vi "Dashboard Main.vi"() -> ()   [LabVIEW 2013]
uses:
  <vilib>/event_ctls.llb/eventvkey.ctl
  <vilib>/Rock Robotics/WPI/Dashboard/WPI_DashboardLogging Global.vi
  <vilib>/Utility/config.llb/Write Key (String).vi
  <vilib>/Utility/config.llb/Write Key (I32).vi
  <vilib>/Utility/config.llb/NI_LVConfig.lvlib
panel:
  out "LED 1":bool
  out "Image Message":string="Timeout in Camera Communications"
  in  "Rec Mode":enum32{"Stop", "Record", "Playback"}(radio)
  in  "Dashboard Tab":T1(tab)
  out "Re-Capture":bool
  out "Ping":dbl
  out "Gauge":dbl(knob) scale=0.0..180.0
  in  "1":dbl=1.0 min=1.0 max=3.0 step=1.0
  in  "Camera Settings":T2={"Frame Rate"=30, "Compression"=30, "Size"=1} {"Frame Rate" scale=1.0..30.0; "Size" items=["640x480", "320x240", "160x120"]}
  out "MotorSliders R":cluster{"MotorSlide1":dbl, "MotorSlide2":dbl} {"MotorSlide2" scale=-1.0..1.0 scale format="%#_2e"; "MotorSlide1" scale=-1.0..1.0 scale format="%#_2e"}
  out "MotorChart R":cluster{"Numeric":dbl, "Numeric":dbl}(graph)
  out "MotorSliders L":T3 {"MotorSlide4 2" scale=0.0..14.0 scale format="%#_2e"; "MotorSlide2" scale=-1.0..1.0 scale format="%#_2e"; "MotorSlide1" scale=-1.0..1.0 scale format="%#_2e"}
  out "MotorChart L":T4(graph)
  out "JS1 Z":dbl(slide) scale=-1.0..1.0 scale format="%#_2e"
  out "Joystick 1":cluster{"X":dbl, "Y":dbl}[](graph)
  out "JS Buttons 1":T5
  out "JS2 Z":dbl(slide) scale=-1.0..1.0 scale format="%#_2e"
  out "Joystick 2":cluster{"X":dbl, "Y":dbl}[](graph)
  out "JS Buttons 2":T5
  out "Mode":T6(ring)=enum."Auto Disabled"
  out "Camera IP":string
  in  "DB Camera Config":bool
  out "fps":dbl format="%#.1g"
  out "Mbps":dbl format="%#.1g"
  out "Mbps 2":bool
  out "Ready to Fire":bool
  out "Vacuum State":bool
  out "Manual":bool
  out "1":bool
  out "2":bool
  out "3":bool
  out "4":bool
  out "Blink":dbl
  out "Ticks":dbl
  out "State Machine State":dbl
  out "State Machine State Name":string
  in  "Slider 1":dbl(slide) scale=0.0..100.0
  in  "Checkbox 2":bool
  in  "Checkbox 1":bool
  in  "Test Slider":dbl(slide) scale=0.0..100.0 scale format="%#_3g"
  in  "On/Off":bool caption="Solenoid"
  in  "Test Name":u16(ring) items=["Select the test to run...", "Example Test", "-------------------------------", "List of tests is built in robot code.", "Replace with your own automated tests."]
  in  "Test Tree":string(tree)
  in  "Motor":cluster{"Value":dbl, "Enable":bool} {"Value" scale=-1.0..1.0 scale format="%#_3g"}
  out "Progress":T7 {"Test Progress" scale=0.0..100.0}
  in  "Rev/Fwd":cluster{"Forward":bool, "Reverse":bool}
  in  "Test Ring":u16(ring) items=["Auto", "Fixed indoor", "Fixed outdoor 1", "Fixed outdoor 2", "Fixed fluorescent 1", "Fixed fluorescent 2", "Hold current"]
  in  "Listbox":i32(listbox)
  out "Tree":string(tree)
  out "Camera Image":T8(plugin-control)
  in  "Enable":bool
  # "Autonomous Presets"
  # "Left"
  # "Front"
  # "Right"
  # "Battery"
  # "Customize by placing controls and indicators here and name to\nmatch Dashboard Variables on robot."
  # "This tab is a great place for autonomous settings and validation.\nCustomize by placing controls and indicators here and name to\nmatch Dashboard Variables on robot."
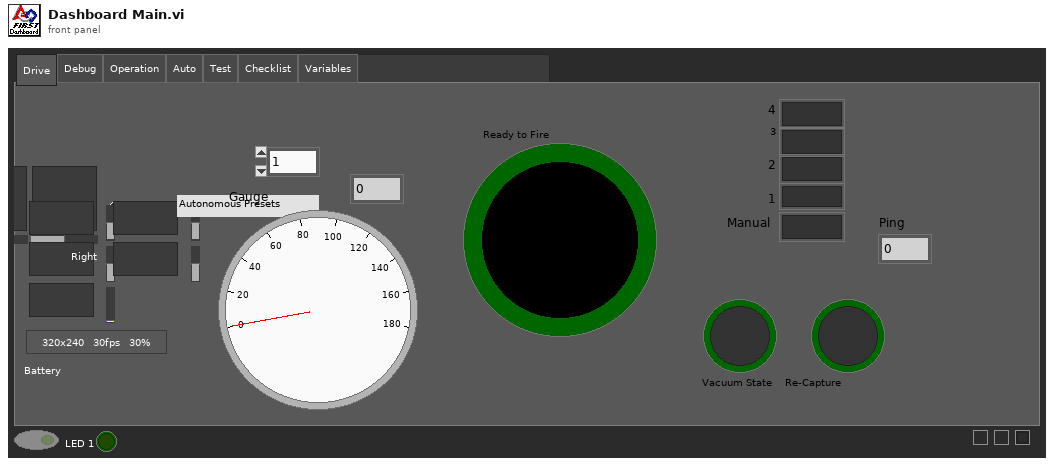
[diagram p1: front panel]
types:
  T1 = enum32{"Drive", "Debug", "Operation", "Auto", "Test", "Checklist", "Variables"}
  T2 = cluster{"Frame Rate":i32, "Compression":i32, "Size":u16}
  T3 = cluster{"MotorSlide1":dbl, "MotorSlide2":dbl, "MotorSlide4 2":dbl}
  T4 = cluster{"Numeric":dbl, "Numeric":dbl, "Battery":sgl}
  T5 = cluster{bool, bool, bool, bool, bool, bool, bool, bool, bool, bool, bool, bool}
  T6 = enum8{"Tele-Op Disabled", "Tele-Op Enabled", "Auto Disabled", "Auto Enabled", "Test Disabled", "Test Enabled", ""}
  T7 = cluster{"Test Progress":u8, "Test Progress Text":string}
  T8 = typedef "IMAQ Image.ctl" = refnum<image>
  T9 = enum32{"Drive", "Operation", "Auto", "Test", "Checklist", "Variables"}
  T10 = typedef "Image Type" = u32
  T11 = cluster{"Digital Inputs":bool[], "Digital Outputs":bool[]}
  T12 = cluster{"Competition mode":bool, "Robot Link":bool, "Autonomous":bool, "Enabled":bool, "E-Stop":bool, "Simulated":bool, "TestMode":bool, "Docked Window":bool}
  T13 = cluster{"Boolean Array[0]":bool, "Boolean Array[1]":bool, "Boolean Array[2]":bool, "Boolean Array[3]":bool, "Boolean Array[4]":bool, "Boolean Array[5]":bool, "Boolean Array[6]":bool, "Boolean Array[7]":bool, "Boolean Array[8]":bool, "Boolean Array[9]":bool, "Boolean Array[10]":bool, "Boolean Array[11]":bool}
  T14 = typedef "NI_LVConfig.lvlib/Config Data RefNum.ctl" = refnum<k1>
  T15 = typedef "eventvkey.ctl" = enum16{"ASCII", "Enter", "Return", "Shift", "Ctrl", "Alt", "Cmd", "Opt", "Caps", "NumLock", "Clear", "Break", "Up", "Down", "Left", "Right", "Insert", "Delete", "Home", "End", "PageUp", "PageDown", "Escape", "Help", "Pause", "ScrollLock", "F1", "F2", "F3", "F4", "F5", "F6", "F7", "F8", "F9", "F10", "F11", "F12", "F13", "F14", "F15", "F16", "F17", "F18", "F19", "F20", "F21", "F22", "F23", "F24", "Play", "VolumeUp", "VolumeDown", "Mute", "Two Byte Char"}
  T16 = cluster{"Image Size":bool, "Image Type":bool, "Pixel Value":bool, "ROI Information":bool, "Zoom Factor":bool}
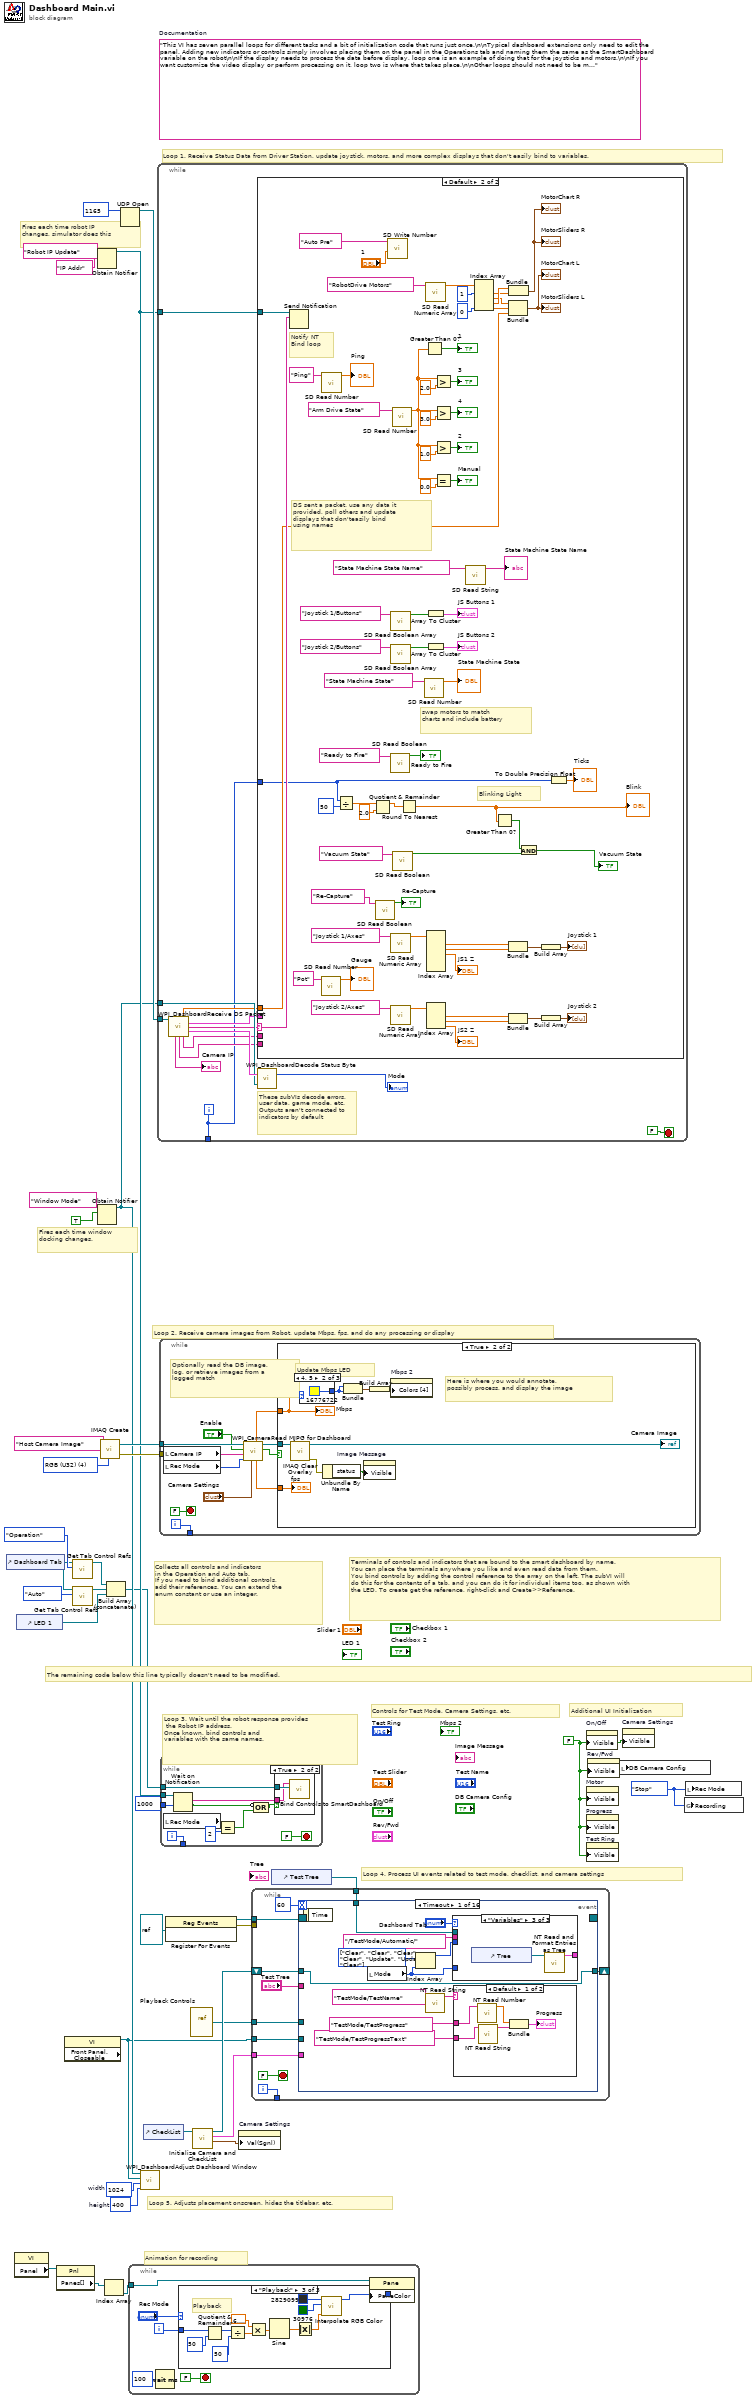
[diagram p0: block diagram]
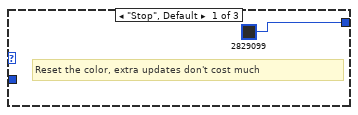
[diagram p2: hidden frame]
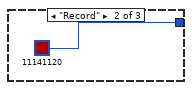
[diagram p3: hidden frame]
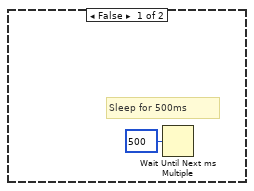
[diagram p5: hidden frame]
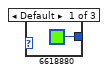
[diagram p6: hidden frame]
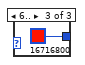
[diagram p7: hidden frame]
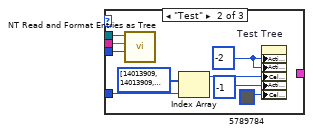
[diagram p9: hidden frame]
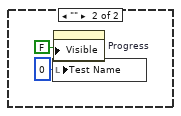
[diagram p10: hidden frame]
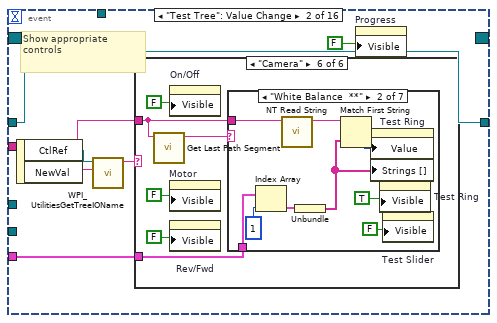
[diagram p11: hidden frame]
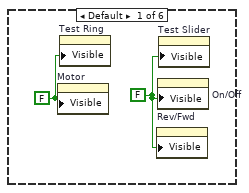
[diagram p12: hidden frame]
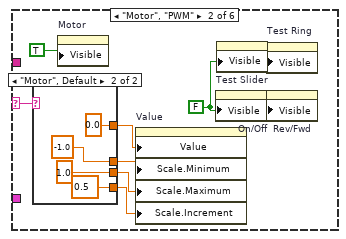
[diagram p13: hidden frame]
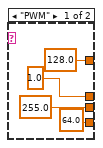
[diagram p14: hidden frame]
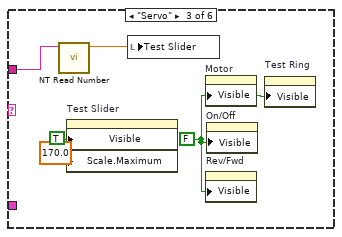
[diagram p15: hidden frame]
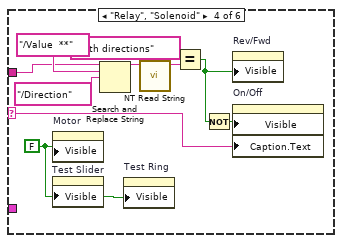
[diagram p16: hidden frame]
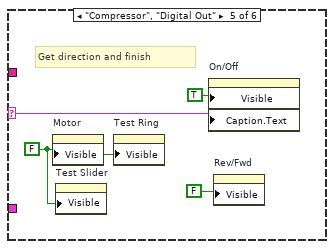
[diagram p17: hidden frame]
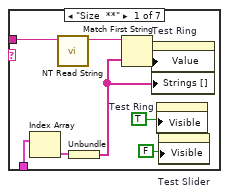
[diagram p18: hidden frame]
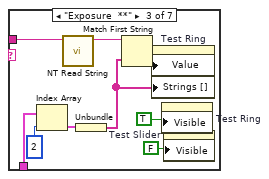
[diagram p19: hidden frame]
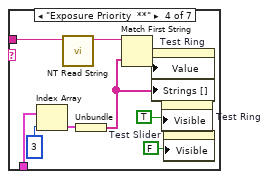
[diagram p20: hidden frame]
diagram:
  w8 = enum32{"Stop", "Record", "Playback"}."Stop" ("Rec Mode")
  w11 = 400  # height
  w12 = 1024  # width
  w25 = FALSE ("Visible")
  (unwired) "This VI has seven parallel loops for different tasks and a bit of initialization code that runs just once.\n\nTypical dashboard extensions only need to edit the panel. Adding new indicators or controls simply involves placing them on the panel in the Operations tab and naming them the same as the SmartDashboard variable on the robot\n\nIf the display needs to process the data before display, loop one is an example of doing that for the joysticks and motors.\n\nIf you want customize the video display or perform processing on it, loop two is where that takes place.\n\nOther loops should not need to be modified. They are pretty standard, and document the task they perform."  # Documentation
  w35 = T10 4 items=["Grayscale (U8)", "Grayscale (I16)", "Grayscale (SGL)", "Complex (CSG)", "RGB (U32)", "HSL (U32)", "RGB (U64)"] ("Image Type")
  # "Controls for Test Mode, Camera Settings, etc."
  # "Additional UI Initialization"
  # "Animation for recording"
  # "Fires each time robot IP\nchanges, simulator does this"
  # "Fires each time window\ndocking changes."
  # "Collects all controls and indicators\nin the Operation and Auto tab.\nIf you need to bind additional controls,\nadd their references. You can extend the\nenum constant or use an integer."
  # "The remaining code below this line typically doesn't need to be modified."
  # "Loop 4. Process UI events related to test mode, checklist, and camera settings"
  # "Terminals of controls and indicators that are bound to the smart dashboard by name.\nYou can place the terminals anywhere you like and even read data from them.\nYou bind controls by adding the control reference to the array on the left. The subVI will\ndo this for the contents of a tab, and you can do it for individual items too, as shown with\nthe LED. To create get the reference, right-click and Create>>Reference."
  # "Loop 3. Wait until the robot response provides\n the Robot IP address.\nOnce known, bind controls and\nvariables with the same names."
  # "Loop 5. Adjusts placement onscreen, hides the titlebar, etc."
  # "Loop 1. Receive Status Data from Driver Station, update joystick, motors, and more complex displays that don't easily bind to variables."
  # "Loop 2. Receive camera images from Robot, update Mbps, fps, and do any processing or display"
  n1 = control-ref of="Dashboard Tab"() -> (w6:refnum<vi>)
  n2 = property class="VI"() -> ("Panel"=w19:refnum<vi>)  [unwired: 2 in, 2 out]
  n3 = control-ref of="LED 1"() -> (w1:refnum<vi>)
  n4 = property class="Pnl"(reference=w19) -> ("Panes[]"=w20:refnum<vi>[])  [unwired: 1 in, 2 out]
  n5 = property class="VI" props=["Front Panel.Closeable"]() -> (reference out=w7:refnum<vi>)  [unwired: 2 in, 2 out]
  n6 = call <vilib>:"Get Tab Control Refs.vi"("Page Index"=T9."Operation" ("Dashboard Tab"), "TabControl in"=w6) -> ("ControlsOnPage"=w4:refnum<vi>[])  [unwired: 9 in]
  n7 = call <vilib>:"Get Tab Control Refs.vi"("Page Index"=T9."Auto" ("Dashboard Tab"), "TabControl in"=w6) -> ("ControlsOnPage"=w5:refnum<vi>[])  [unwired: 9 in]
  n8 = Obtain Notifier(name (unnamed)="Robot IP Update", notification data type="IP Addr" ("name (unnamed)")) -> (notifier out=w29:refnum<notifier>)  [unwired: 2 in, 2 out]
  n9 = Obtain Notifier(name (unnamed)="Window Mode", notification data type=TRUE) -> (notifier out=w10:refnum<notifier>)  [unwired: 2 in, 2 out]
  n10 = call "IMAQ Create"("Image Name"="Host Camera Image", "Image Type"=w35) -> ("New Image"=w33:T8, "error out"=w32:errorcluster)  [unwired: 2 in, 1 out]
  n11 = Index Array(array=w20) -> (element=w18:refnum<vi>)  [unwired: 1 in]
  n12 = Build Array (concatenate)(w4, w5, w1) -> (w3:refnum<vi>[])
  n13 = UDP Open(11:u16 1165 ("port")) -> (port=w36:refnum<k16>)  [unwired: 2 in, 4 out]
  n14 = while {
    tunnel: w18 -> [w39]
    i -> [w42]
    stop <- FALSE stop-if-true
    n15 = Wait (ms)(milliseconds to wait=u32 100) -> ()  [unwired: 1 out]
    n16 = case shown="\"Playback\"" "Rec Mode" {
      tunnel: w42 -> [_ _ w57]
      tunnel: [u32 2829099 ("Base Color") u32 11141120 ("Target Color") w46] -> w38
      frame "Stop", Default {
        # "Reset the color, extra updates don't cost much"
      }
      frame "Record" {
      }
      frame "Playback" {
        # "Playback"
        n17 = Quotient & Remainder(x=w57, y=u32 50 ("milliseconds to wait")) -> (x-y*floor(x/y)=w53:u32)  [unwired: 1 out]
        n18 = Divide(x=w53, y=u32 50 ("milliseconds to wait")) -> (x/y=w50:dbl)
        n19 = Multiply(x=6.283185307179586, y=w50) -> (x*y=w55:dbl)
        n20 = Sine(x=w55) -> (sin(x)=w54:dbl)
        n21 = Absolute Value(x=w54) -> (abs(x)=w47:dbl)
        n22 = call "Interpolate RGB Color.vi"("Proportion"=w47, "Target Color"=u32 30976, "Base Color"=u32 2829099) -> ("Result Color"=w46:u32)  [unwired: 8 in]
      }
    }
    n23 = property class="Pane"(reference=w39, "PaneColor"=w38) -> ()  [unwired: 1 in, 2 out]
  }
  n24 = call <vilib>:"WPI_DashboardAdjust Dashboard Window.vi"("height"=w11, "width"=w12, "reference in"=w7, "Notifier in"=w10) -> ()  [unwired: 8 in]
  n25 = control-ref of="CheckList"() -> (w9:refnum<vi>)
  n26 = while {
    tunnel: w36 -> [w68]
    tunnel: w29 -> [w64]
    tunnel: w10 -> [w67]
    tunnel: [w58] -> _
    i -> [w58]
    stop <- FALSE stop-if-true
    # "These subVIs decode errors, user data, game mode, etc.\nOutputs aren't connected to indicators by default"
    n27 = call <vilib>:"WPI_DashboardReceive DS Packet.vi"("Recv Socket"=w68) -> ("Battery"=w59:sgl, "Driver Station"=w60:T11, "Robot IP Address"=w63:string, "Status"=w69:T12, "Camera IP Address"=→"Camera IP":string, "Low Priority User Data"=w62:string, "High Priority User Data"=w61:string)  [unwired: 1 in, 7 out]
    n28 = case shown="Default" w63 {
      selector: w63 -> [_ w117]
      tunnel: w64 -> [_ w118]
      tunnel: w62 -> [_ _]
      tunnel: w61 -> [_ _]
      tunnel: w60 -> [_ _]
      tunnel: w59 -> [_ w116]
      tunnel: w58 -> [_ w77]
      frame "0.0.0.0" {
        # "DS not sending packets, or no robot exists yet.\nDon't poll the variables"
      }
      frame Default {
        # "Blinking Light"
        # "Notify NT\nBind loop"
        # "DS sent a packet. use any data it\nprovided, poll others and update\ndisplays that don'teasily bind\nusing names"
        # "swap motors to match\ncharts and include battery"
        n29 = Send Notification(notification=w117, notifier=w118) -> ()  [unwired: 1 in, 2 out]
        n30 = call <vilib>:"SD Read Number.vi"("Name"="Pot") -> ("Numeric"=→"Gauge":dbl)  [unwired: 8 in, 2 out]
        n31 = call <vilib>:"SD Read Number.vi"("Name"="Ping") -> ("Numeric"=→"Ping":dbl)  [unwired: 8 in, 2 out]
        n32 = Divide(x=w77, y=50) -> (x/y=w79:dbl)
        n33 = Quotient & Remainder(x=w79, y=2.0) -> (x-y*floor(x/y)=w75:dbl)  [unwired: 1 out]
        n34 = call <vilib>:"SD Read Boolean.vi"("Name"="Re-Capture") -> ("Boolean"=→"Re-Capture":bool)  [unwired: 8 in, 2 out]
        n35 = call <vilib>:"SD Write Number.vi"("Numeric"="1", "Name"="Auto Pre") -> ()  [unwired: 8 in, 2 out]
        n36 = call <vilib>:"SD Read Boolean.vi"("Name"="Ready to Fire") -> ("Boolean"=→"Ready to Fire":bool)  [unwired: 8 in, 2 out]
        n37 = call <vilib>:"SD Read Boolean Array.vi"("Name"="Joystick 1/Buttons") -> ("Boolean Array"=w136:bool[])  [unwired: 8 in, 2 out]
        n38 = call <vilib>:"SD Read Boolean Array.vi"("Name"="Joystick 2/Buttons") -> ("Boolean Array"=w127:bool[])  [unwired: 8 in, 2 out]
        n39 = call <vilib>:"SD Read Numeric Array.vi"("Name"="Joystick 1/Axes") -> ("Numeric Array"=w134:dbl[])  [unwired: 8 in, 2 out]
        n40 = call <vilib>:"SD Read Numeric Array.vi"("Name"="Joystick 2/Axes") -> ("Numeric Array"=w128:dbl[])  [unwired: 8 in, 2 out]
        n41 = call <vilib>:"SD Read Number.vi"("Name"="Arm Drive State") -> ("Numeric"=w96:dbl)  [unwired: 8 in, 2 out]
        n42 = call <vilib>:"SD Read Boolean.vi"("Name"="Vacuum State") -> ("Boolean"=w72:bool)  [unwired: 8 in, 2 out]
        n43 = Round To Nearest(number=w75) -> (nearest integer value=w74:dbl)
        "Blink" <- w74
        n44 = call <vilib>:"SD Read Number.vi"("Name"="State Machine State") -> ("Numeric"=→"State Machine State":dbl)  [unwired: 8 in, 2 out]
        n45 = Greater Than 0?(x=w96) -> (x > 0?=→"1":bool)
        n46 = call <vilib>:"SD Read Numeric Array.vi"("Name"="RobotDrive Motors") -> ("Numeric Array"=w115:dbl[])  [unwired: 8 in, 2 out]
        n47 = Array To Cluster(array=w136) -> (cluster=→"JS Buttons 1":T13)
        n48 = Array To Cluster(array=w127) -> (cluster=→"JS Buttons 2":T13)
        n49 = Index Array(array=w134) -> (element #1=w131:dbl, element #2=w132:dbl, element #3=→"JS1 Z":dbl)  [unwired: 6 in, 3 out]
        n50 = Index Array(array=w128) -> (element #1=w123:dbl, element #2=w122:dbl, element #3=→"JS2 Z":dbl)  [unwired: 3 in]
        n51 = Greater?(x=w96, y=2.0) -> (0:→"3":bool)
        n52 = Greater?(x=w96, y=3.0) -> (0:→"4":bool)
        n53 = Greater?(x=w96, y=1.0) -> (0:→"2":bool)
        n54 = Equal?(x=w96, y=0.0) -> (x = y?=→"Manual":bool)
        n55 = call <vilib>:"SD Read String.vi"("Name"="State Machine State Name") -> ("String"=→"State Machine State Name":string)  [unwired: 8 in, 2 out]
        n56 = Index Array(array=w115, index #1=1, index #4=0) -> (element #1=w111:dbl, element #2=w110:dbl, element #3=w112:dbl, element #4=w107:dbl)  [unwired: 2 in]
        n57 = Greater Than 0?(x=w74) -> (x > 0?=w73:bool)
        n58 = Bundle("Numeric"=w110, "Numeric"=w107, "Battery"=w116) -> (→"MotorChart L" →"MotorSliders L":T4)  [unwired: 1 in]
        n59 = Bundle("Numeric"=w131, "Numeric"=w132) -> (w130:cluster{"Numeric":dbl, "Numeric":dbl})  [unwired: 1 in]
        n60 = Bundle("Numeric"=w123, "Numeric"=w122) -> (w124:cluster{"Numeric":dbl, "Numeric":dbl})  [unwired: 1 in]
        n61 = Bundle("Numeric"=w112, "Numeric"=w111) -> (→"MotorChart R" →"MotorSliders R":cluster{"Numeric":dbl, "Numeric":dbl})  [unwired: 1 in]
        n62 = And(x=w73, y=w72) -> (x .and. y?=→"Vacuum State":bool)
        n63 = Build Array(w130) -> (→"Joystick 1":cluster{"Numeric":dbl, "Numeric":dbl}[])
        n64 = Build Array(w124) -> (→"Joystick 2":cluster{"Numeric":dbl, "Numeric":dbl}[])
        n65 = To Double Precision Float(number=w77) -> (double precision float=→"Ticks":dbl)
      }
    }
    n66 = call <vilib>:"WPI_DashboardDecode Status Byte.vi"("Window Mode Notifier"=w67, "Status"=w69) -> ("Mode"=→"Mode":T6)  [unwired: 1 out]
  }
  n67 = while {
    tunnel: w33 -> [w148]
    tunnel: w32 -> [_]
    tunnel: [w149] -> _
    i -> [w149]
    stop <- FALSE stop-if-true
    # "Optionally read the DB image,\nlog, or retrieve images from a\nlogged match"
    n68 = local read "Camera IP"() -> (w141:string)
    n69 = local read "Rec Mode"() -> (w140:enum32{"Stop", "Record", "Playback"})
    n70 = call <vilib>:"WPI_CameraRead MJPG for Dashboard.vi"("Camera Settings"="Camera Settings", "Rec Mode"=w140, "Camera IP"=w141, "Enable"="Enable", "Refnum in"=w148) -> ("Active"=w145:bool, "Refnum out"=w147:T8, "FPS"=w144:dbl, "Bandwidth (Mbps)"=w143:dbl)  [unwired: 3 in]
    n71 = case shown="True" w145 {
      tunnel: w147 -> [_ w155]
      tunnel: w143 -> [_ w154]
      tunnel: w144 -> [_ w152]
      frame False {
        # "Sleep for 500ms"
        n72 = Wait Until Next ms Multiple(millisecond multiple=u32 500) -> ()  [unwired: 1 out]
      }
      frame True {
        # "Here is where you would annotate,\npossibly process, and display the image"
        # "Update Mbps LED"
        n73 = call "IMAQ Clear Overlay"("Image"=w155) -> ("error out"=w159:errorcluster, "Image Out"=→"Camera Image":T8)  [unwired: 2 in, 7 out]
        n74 = case shown="4, 5" w154 {
          tunnel: [u32 6618880 ("Color Box") u32 16776722 ("Color Box") u32 16716800 ("Color Box")] -> w156
          frame Default {
          }
          frame 4, 5 {
          }
          frame 6.. {
          }
        }
        n75 = Unbundle By Name(w159) -> ("status"=w160:bool)
        n76 = Bundle("Color Box"=w156, "Color Box"=w156) -> (w158:cluster{"Color Box":u32, "Color Box":u32})  [unwired: 1 out]
        n77 = property on="Image Message" class="Str"("Visible"=w160) -> ()  [unwired: 2 in, 2 out]
        n78 = Build Array(w158) -> (w157:cluster{"Color Box":u32, "Color Box":u32}[])
        n79 = property on="Mbps 2" class="Bool (strict)"("Colors [4]"=w157) -> ()  [unwired: 2 in, 2 out]
        "Mbps" <- w154
        "fps" <- w152
      }
    }
  }
  n80 = while {
    tunnel: w3 -> [w174]
    tunnel: w29 -> [w172]
    tunnel: [w170] -> _
    tunnel: u32 1000 ("milliseconds to wait") -> [w169]
    i -> [w170]
    stop <- FALSE stop-if-true
    n81 = local read "Rec Mode"() -> (w165:enum32{"Stop", "Record", "Playback"})
    n82 = Wait on Notification(notifier=w172, timeout in ms (-1)=w169) -> (notification=w171:string, timed out?=w167:bool)  [unwired: 2 in, 2 out]
    n83 = Equal?(x=w165, y=u16 2 ("Rec Mode")) -> (x = y?=w166:bool)
    n84 = Compound Arithmetic op=OR(invert w167, w166) -> (w168:bool)
    n85 = case shown="True" w168 {
      tunnel: w174 -> [_ w176]
      tunnel: w171 -> [_ w175]
      frame False {
      }
      frame True {
        n86 = call <vilib>:"Bind Controls to SmartDashboard.vi"("Bound Control Refs"=w176, "Server IP Address"=w175) -> ()  [unwired: 10 in]
      }
    }
  }
  n87 = register-events(refnum<vi> refnum) -> (reference out=w16:refnum<event-registration>, error out=w15:errorcluster)  [unwired: 2 in]
  n88 = vi-ref "Playback Controls.vi"() -> (w17:refnum<vi>)
  n89 = call "Initialize Camera and CheckList.vi"("ListBox in"=w9) -> ("Cluster"=w23:cluster{"value":i32, "value":i32, "index":i32}, "Array"=w24:cluster{string[]}[], "File Refnum"=w22:T14)  [unwired: 8 in]
  n90 = property on="Camera Settings" class="Clust (strict)"("Val(Sgnl)"=w23) -> ()  [unwired: 2 in, 2 out]
  n91 = control-ref of="Test Tree"() -> (w21:refnum<vi>)
  n92 = while {
    tunnel: w24 -> [w184]
    shift-right: [w183] -> _
    shift-left: w22 -> [w182]
    tunnel: [w181] -> _
    tunnel: w21 -> [w180]
    tunnel: w17 -> [w179]
    tunnel: w16 -> [w178]
    tunnel: w15 -> [_]
    tunnel: w7 -> [w177]
    i -> [w181]
    stop <- FALSE stop-if-true
    n93 = event shown="[0] Timeout" {
      selector: w178 -> [_ _ _ _ _ _ _ _ _ _ _ _ _ _ _ _]
      dyn-events: [_ _ _ _ _ _ _ _ _ _ _ _ _ w422 _ _] -> _
      timeout: u32 60 ("milliseconds to wait") -> [_ _ _ _ _ _ _ _ _ _ _ _ _ _ _ _]
      tunnel: w180 -> [w194 _ _ _ _ _ _ _ _ _ _ _ _ _ _ _]
      tunnel: "Test Tree" -> [_ _ _ _ _ _ _ _ w391 w399 w401 w405 w413 _ _ _]
      tunnel: w184 -> [_ w218 _ _ _ _ w355 w385 _ _ _ _ _ _ _ _]
      tunnel: [w188 w217 w316 w321 w329 w341 w354 w378 w390 w397 w400 w404 w412 w424 w438 w439] -> w183
      tunnel: w182 -> [w188 w217 w316 w321 w329 w341 w353 w378 w390 w397 w400 w404 w412 w424 w438 w439]
      tunnel: w179 -> [_ _ _ _ _ _ _ _ _ _ _ _ _ w425 _ w442]
      tunnel: w177 -> [_ _ _ _ _ _ _ _ _ _ _ _ _ w420 _ _]
      event Timeout {
        w193 = enum16{"Update", "Clear"}[] [enum."Clear", enum."Clear", enum."Clear", enum."Clear", enum."Update", enum."Update", enum."Clear"] items=["Update", "Clear"]
        n94 = event-data() -> ()  [unwired: 1 in, 1 out]
        n95 = local read "Mode"() -> (w191:T6)
        n96 = Index Array(array=w193, index=w191) -> (element=w192:enum16{"Update", "Clear"})
        n97 = call <vilib>:"NT Read String.vi"("Name"="TestMode/TestName") -> ("String"=w197:string)  [unwired: 9 in, 1 out]
        n98 = case shown="\"Variables\"" "Dashboard Tab" {
          tunnel: w194 -> [_ w207 _]
          tunnel: "/TestMode/Automatic/" ("Name Pattern") -> [_ w206 _]
          tunnel: w192 -> [_ w205 _]
          tunnel: w191 -> [_ w203 _]
          tunnel: [_ _ w209] -> _
          frame "Operation", Default {
          }
          frame "Test" {
            w202 = -2 ("Active Item:Row Number")
            n99 = call <vilib>:"NT Read and Format Entries as Tree.vi"("Operation"=w205, "Name Pattern"=w206, "Tree Refnum"=w207) -> ()  [unwired: 7 in, 2 out]
            n100 = Index Array(array=u32[] [14013909, 14013909, 14013909, 14013909, 14013909, 16777215, 14013909], index=w203) -> (element=w201:u32)
            n101 = property on="Test Tree" class="Tree (strict)"("Active Item Row Number"=w202, "ActiveColNum"=w202, "CellBG"=w201, "Active Item Row Number"=-1 ("Active Item:Row Number"), "CellBG"=u32 5789784 ("Color Box")) -> ()  [unwired: 2 in, 2 out]
          }
          frame "Variables" {
            n102 = control-ref of="Tree"() -> (w208:refnum<vi>)
            n103 = call <vilib>:"NT Read and Format Entries as Tree.vi"("Tree Refnum"=w208) -> ("Formatted Strings"=w209:cluster{"Name":string, "Value":string}[])  [unwired: 9 in, 1 out]
          }
        }
        n104 = case shown="Default" w197 {
          tunnel: "TestMode/TestProgress" ("Name") -> [w211 _]
          tunnel: "TestMode/TestProgressText" ("Name") -> [w210 _]
          frame Default {
            n105 = call <vilib>:"NT Read Number.vi"("Name"=w211) -> ("Numeric"=w212:dbl)  [unwired: 9 in, 1 out]
            n106 = call <vilib>:"NT Read String.vi"("Name"=w210) -> ("String"=w213:string)  [unwired: 9 in, 1 out]
            n107 = Bundle("Numeric"=w212, "String"=w213) -> (→"Progress":cluster{"Numeric":dbl, "String":string})  [unwired: 1 in]
          }
          frame "" {
            n108 = local write "Test Name"(u16 0) -> ()
            n109 = property on="Progress" class="Clust (strict)"("Visible"=FALSE) -> ()  [unwired: 2 in, 2 out]
          }
        }
      }
      event "Test Tree": Value Change {
        # "Show appropriate\ncontrols"
        n110 = event-data() -> ("CtlRef"=w221:refnum<vi>, "NewVal"=w219:string)  [unwired: 1 in]
        n111 = call <vilib>:"WPI_UtilitiesGetTreeIOName.vi"("NewVal"=w219, "TreeControl in"=w221) -> ("I/O Name"=w222:string)  [unwired: 9 in]
        n112 = case shown="\"Camera\"" w222 {
          selector: w222 -> [_ w229 _ w247 w256 _]
          tunnel: w219 -> [_ _ w244 w246 _ w263]
          tunnel: w218 -> [_ _ _ _ _ w262]
          frame Default {
            w224 = FALSE ("Visible")
            w223 = FALSE ("Visible")
            n113 = property on="Motor" class="Clust (strict)"("Visible"=w223) -> ()  [unwired: 2 in, 2 out]
            n114 = property on="Test Ring" class="Ring (strict)"("Visible"=w223) -> ()  [unwired: 2 in, 2 out]
            n115 = property on="Rev/Fwd" class="Clust (strict)"("Visible"=w224) -> ()  [unwired: 2 in, 2 out]
            n116 = property on="On/Off" class="Bool (strict)"("Visible"=w224) -> ()  [unwired: 2 in, 2 out]
            n117 = property on="Test Slider" class="Slide (strict)"("Visible"=w224) -> ()  [unwired: 2 in, 2 out]
          }
          frame "Motor", "PWM" {
            w230 = FALSE ("Visible")
            n118 = case shown="\"Motor\", Default" w229 {
              tunnel: [1.0 ("Value") -1.0 ("Value")] -> w228
              tunnel: [255.0 ("Value") 1.0 ("Value")] -> w227
              tunnel: [128.0 ("Value") 0.0 ("Value")] -> w226
              tunnel: [64.0 ("Value") 0.5 ("Value")] -> w225
              frame "PWM" {
              }
              frame "Motor", Default {
              }
            }
            n119 = property on="Motor" class="Clust (strict)"("Visible"=TRUE) -> ()  [unwired: 2 in, 2 out]
            n120 = property on="Value" class="Slide (strict)"("Value"=w226, "Scale.Minimum"=w228, "Scale.Maximum"=w227, "Scale.Increment"=w225) -> ()  [unwired: 2 in, 2 out]
            n121 = property on="On/Off" class="Bool (strict)"("Visible"=w230) -> ()  [unwired: 2 in, 2 out]
            n122 = property on="Test Slider" class="Slide (strict)"("Visible"=w230) -> ()  [unwired: 2 in, 2 out]
            n123 = property on="Test Ring" class="Ring (strict)"("Visible"=w230) -> ()  [unwired: 2 in, 2 out]
            n124 = property on="Rev/Fwd" class="Clust (strict)"("Visible"=w230) -> ()  [unwired: 2 in, 2 out]
          }
          frame "Servo" {
            w242 = FALSE ("Visible")
            n125 = call <vilib>:"NT Read Number.vi"("Name"=w244) -> ("Numeric"=w243:dbl)  [unwired: 9 in, 1 out]
            n126 = property on="Test Slider" class="Slide (strict)"("Visible"=TRUE, "Scale.Maximum"=170.0 ("Scale.Range:Maximum")) -> ()  [unwired: 2 in, 2 out]
            n127 = local write "Test Slider"(w243) -> ()
            n128 = property on="Motor" class="Clust (strict)"("Visible"=w242) -> ()  [unwired: 2 in, 2 out]
            n129 = property on="Rev/Fwd" class="Clust (strict)"("Visible"=w242) -> ()  [unwired: 2 in, 2 out]
            n130 = property on="On/Off" class="Bool (strict)"("Visible"=w242) -> ()  [unwired: 2 in, 2 out]
            n131 = property on="Test Ring" class="Ring (strict)"("Visible"=w242) -> ()  [unwired: 2 in, 2 out]
          }
          frame "Relay", "Solenoid" {
            w245 = FALSE ("Visible")
            n132 = property on="Motor" class="Clust (strict)"("Visible"=w245) -> ()  [unwired: 2 in, 2 out]
            n133 = property on="Test Slider" class="Slide (strict)"("Visible"=w245) -> ()  [unwired: 2 in, 2 out]
            n134 = Search and Replace String(input string=w246, search string="/Value  **", replace string="/Direction") -> (result string=w252:string)  [unwired: 5 in, 3 out]
            n135 = property on="Test Ring" class="Ring (strict)"("Visible"=w245) -> ()  [unwired: 2 in, 2 out]
            n136 = call <vilib>:"NT Read String.vi"("Name"=w252) -> ("String"=w250:string)  [unwired: 9 in, 1 out]
            n137 = Equal?(x="Both directions", y=w250) -> (x = y?=w248:bool)
            n138 = Not(x=w248) -> (.not. x?=w249:bool)
            n139 = property on="Rev/Fwd" class="Clust (strict)"("Visible"=w248) -> ()  [unwired: 2 in, 2 out]
            n140 = property on="On/Off" class="Bool (strict)"("Visible"=w249, "Caption.Text"=w247) -> ()  [unwired: 2 in, 2 out]
          }
          frame "Compressor", "Digital Out" {
            w255 = FALSE ("Visible")
            # "Get direction and finish"
            n141 = property on="Motor" class="Clust (strict)"("Visible"=w255) -> ()  [unwired: 2 in, 2 out]
            n142 = property on="Test Slider" class="Slide (strict)"("Visible"=w255) -> ()  [unwired: 2 in, 2 out]
            n143 = property on="Test Ring" class="Ring (strict)"("Visible"=w255) -> ()  [unwired: 2 in, 2 out]
            n144 = property on="On/Off" class="Bool (strict)"("Visible"=TRUE, "Caption.Text"=w256) -> ()  [unwired: 2 in, 2 out]
            n145 = property on="Rev/Fwd" class="Clust (strict)"("Visible"=FALSE) -> ()  [unwired: 2 in, 2 out]
          }
          frame "Camera" {
            n146 = call <vilib>:"Get Last Path Segment.vi"("String in"=w263) -> ("String out"=w264:string)  [unwired: 10 in]
            n147 = property on="On/Off" class="Bool (strict)"("Visible"=FALSE) -> ()  [unwired: 2 in, 2 out]
            n148 = property on="Motor" class="Clust (strict)"("Visible"=FALSE) -> ()  [unwired: 2 in, 2 out]
            n149 = property on="Rev/Fwd" class="Clust (strict)"("Visible"=FALSE) -> ()  [unwired: 2 in, 2 out]
            n150 = case shown="\"White Balance  **\"" w264 {
              tunnel: w263 -> [w270 w279 w288 w297 w306 _ w312]
              tunnel: w262 -> [w268 w276 w285 w294 w303 _ _]
              frame "Size  **" {
                n151 = Index Array(array=w268) -> (element=w267:cluster{string[]})  [unwired: 1 in]
                n152 = call <vilib>:"NT Read String.vi"("Name"=w270) -> ("String"=w269:string)  [unwired: 9 in, 1 out]
                n153 = Unbundle(w267) -> (w265:string[])
                n154 = Match First String(2:w265, 3:w269) -> (0:w266:i32)  [unwired: 1 out]
                n155 = property on="Test Ring" class="Ring (strict)"("Value"=w266, "Strings []"=w265) -> ()  [unwired: 2 in, 2 out]
                n156 = property on="Test Ring" class="Ring (strict)"("Visible"=TRUE) -> ()  [unwired: 2 in, 2 out]
                n157 = property on="Test Slider" class="Slide (strict)"("Visible"=FALSE) -> ()  [unwired: 2 in, 2 out]
              }
              frame "White Balance  **" {
                n158 = Index Array(array=w276, index=1) -> (element=w277:cluster{string[]})
                n159 = call <vilib>:"NT Read String.vi"("Name"=w279) -> ("String"=w278:string)  [unwired: 9 in, 1 out]
                n160 = Unbundle(w277) -> (w274:string[])
                n161 = Match First String(2:w274, 3:w278) -> (0:w273:i32)  [unwired: 1 out]
                n162 = property on="Test Ring" class="Ring (strict)"("Value"=w273, "Strings []"=w274) -> ()  [unwired: 2 in, 2 out]
                n163 = property on="Test Ring" class="Ring (strict)"("Visible"=TRUE) -> ()  [unwired: 2 in, 2 out]
                n164 = property on="Test Slider" class="Slide (strict)"("Visible"=FALSE) -> ()  [unwired: 2 in, 2 out]
              }
              frame "Exposure  **" {
                n165 = Index Array(array=w285, index=2) -> (element=w286:cluster{string[]})
                n166 = call <vilib>:"NT Read String.vi"("Name"=w288) -> ("String"=w287:string)  [unwired: 9 in, 1 out]
                n167 = Unbundle(w286) -> (w282:string[])
                n168 = Match First String(2:w282, 3:w287) -> (0:w283:i32)  [unwired: 1 out]
                n169 = property on="Test Ring" class="Ring (strict)"("Value"=w283, "Strings []"=w282) -> ()  [unwired: 2 in, 2 out]
                n170 = property on="Test Ring" class="Ring (strict)"("Visible"=TRUE) -> ()  [unwired: 2 in, 2 out]
                n171 = property on="Test Slider" class="Slide (strict)"("Visible"=FALSE) -> ()  [unwired: 2 in, 2 out]
              }
              frame "Exposure Priority  **" {
                n172 = Index Array(array=w294, index=3) -> (element=w295:cluster{string[]})
                n173 = call <vilib>:"NT Read String.vi"("Name"=w297) -> ("String"=w296:string)  [unwired: 9 in, 1 out]
                n174 = Unbundle(w295) -> (w291:string[])
                n175 = Match First String(2:w291, 3:w296) -> (0:w292:i32)  [unwired: 1 out]
                n176 = property on="Test Ring" class="Ring (strict)"("Value"=w292, "Strings []"=w291) -> ()  [unwired: 2 in, 2 out]
                n177 = property on="Test Ring" class="Ring (strict)"("Visible"=TRUE) -> ()  [unwired: 2 in, 2 out]
                n178 = property on="Test Slider" class="Slide (strict)"("Visible"=FALSE) -> ()  [unwired: 2 in, 2 out]
              }
              frame "Color Enable  **" {
                n179 = Index Array(array=w303, index=4) -> (element=w304:cluster{string[]})
                n180 = call <vilib>:"NT Read String.vi"("Name"=w306) -> ("String"=w305:string)  [unwired: 9 in, 1 out]
                n181 = Unbundle(w304) -> (w300:string[])
                n182 = Match First String(2:w300, 3:w305) -> (0:w301:i32)  [unwired: 1 out]
                n183 = property on="Test Ring" class="Ring (strict)"("Value"=w301, "Strings []"=w300) -> ()  [unwired: 2 in, 2 out]
                n184 = property on="Test Ring" class="Ring (strict)"("Visible"=TRUE) -> ()  [unwired: 2 in, 2 out]
                n185 = property on="Test Slider" class="Slide (strict)"("Visible"=FALSE) -> ()  [unwired: 2 in, 2 out]
              }
              frame Default {
                n186 = property on="Test Ring" class="Ring (strict)"("Visible"=FALSE) -> ()  [unwired: 2 in, 2 out]
                n187 = property on="Test Slider" class="Slide (strict)"("Visible"=FALSE) -> ()  [unwired: 2 in, 2 out]
              }
              frame "Brightness  **", "Color Level  **", "Compression  **", "FPS  **", "Sharpness  **" {
                n188 = call <vilib>:"NT Read Number.vi"("Name"=w312) -> ("Numeric"=w311:dbl)  [unwired: 9 in, 1 out]
                n189 = local write "Test Slider"(w311) -> ()
                n190 = property on="Test Slider" class="Slide (strict)"("Visible"=TRUE, "Scale.Maximum"=100.0 ("Scale.Range:Maximum")) -> ()  [unwired: 2 in, 2 out]
                n191 = property on="Test Ring" class="Ring (strict)"("Visible"=FALSE) -> ()  [unwired: 2 in, 2 out]
              }
            }
          }
        }
        n192 = property on="Progress" class="Clust (strict)"("Visible"=FALSE) -> ()  [unwired: 2 in, 2 out]
      }
      event "Test Name": Mouse Enter {
        # "Populate the ring with the list of tests"
        n193 = event-data() -> ()  [unwired: 1 in, 1 out]
        n194 = call <vilib>:"NT Read String Array.vi"("Name"="TestMode/TestList") -> ("String Array"=w320:string[])  [unwired: 9 in, 1 out]
        n195 = Build Array (concatenate)("Select the test to run...", w320) -> (w319:string[])
        n196 = property on="Test Name" class="Ring (strict)"("Strings []"=w319) -> ()  [unwired: 2 in, 2 out]
      }
      event "Test Name": Value Change {
        w322 = FALSE ("Visible")
        # "Tell the robot the test name to run"
        n197 = event-data() -> ("NewVal"=w326:u16)  [unwired: 1 in]
        n198 = property on="Test Name" class="Ring (strict)"() -> ("Strings []"=w327:string[])  [unwired: 2 in, 2 out]
        n199 = local write "Progress"(T7 {"Test Progress"=0, "Test Progress Text"=""} ("Progress")) -> ()
        n200 = Index Array(array=w327, index=w326) -> (element=w325:string)
        n201 = call <vilib>:"NT Write String.vi"("String"=w325, "Name"="TestMode/TestName") -> ()  [unwired: 9 in, 1 out]
        n202 = property on="Progress" class="Clust (strict)"("Visible"=TRUE) -> ()  [unwired: 2 in, 2 out]
        n203 = property on="Motor" class="Clust (strict)"("Visible"=w322) -> ()  [unwired: 2 in, 2 out]
        n204 = property on="Test Slider" class="Slide (strict)"("Visible"=w322) -> ()  [unwired: 2 in, 2 out]
        n205 = property on="On/Off" class="Bool (strict)"("Visible"=w322) -> ()  [unwired: 2 in, 2 out]
        n206 = property on="Rev/Fwd" class="Clust (strict)"("Visible"=w322) -> ()  [unwired: 2 in, 2 out]
        n207 = property on="Test Ring" class="Ring (strict)"("Visible"=w322) -> ()  [unwired: 2 in, 2 out]
      }
      event "Listbox": Double Click {
        n208 = event-data() -> ("PlatMods.Shift"=w330:bool, "Row"=w332:i32)  [unwired: 1 in]
        n209 = case shown="True" w330 {
          tunnel: w332 -> [w336 _]
          tunnel: 1 -> [w335 _]
          frame False {
            n210 = property on="Listbox" class="LstBox (strict)"() -> ("Item Symbols"=w334:i32[])  [unwired: 2 in, 2 out]
            n211 = Replace Array Subset(array=w334, new element=w335, index=w336) -> (w333:i32[])
            n212 = property on="Listbox" class="LstBox (strict)"("Item Symbols"=w333) -> ()  [unwired: 2 in, 2 out]
          }
          frame True {
            w337 = 0 ("Top Row")
            n213 = property on="Listbox" class="LstBox (strict)"() -> ("Number of Rows"=w339:u32)  [unwired: 2 in, 2 out]
            n214 = Initialize Array(0, w339) -> (w338:i32[])
            n215 = property on="Listbox" class="LstBox (strict)"("Top Row"=w337, "Value"=w337, "Item Symbols"=w338) -> ()  [unwired: 2 in, 2 out]
          }
        }
      }
      event "Listbox": Key Down {
        n216 = event-data() -> ("VKey"=w343:T15)  [unwired: 1 in]
        n217 = case shown="\"Left\", \"Right\"" w343 {
          selector: w343 -> [w348 _]
          tunnel: eventvkey."Left" ("VKey") -> [w346 _]
          frame "Left", "Right" {
            n218 = Equal?(x=w346, y=w348) -> (x = y?=w347:bool)
            n219 = Select(t=0, s=w347, f=1) -> (s? t:f=w349:i32)
            n220 = property on="Listbox" class="LstBox (strict)"() -> ("Item Symbols"=w352:i32[])  [unwired: 2 in, 2 out]
            n221 = Replace Array Subset(array=w352, new element=w349, index="Listbox") -> (w351:i32[])
            n222 = property on="Listbox" class="LstBox (strict)"("Item Symbols"=w351) -> ()  [unwired: 2 in, 2 out]
          }
          frame Default {
          }
        }
      }
      event "DB Camera Config": Value Change {
        n223 = event-data() -> ("NewVal"=w356:bool)  [unwired: 1 in]
        n224 = case shown="False" w356 {
          tunnel: w355 -> [w365 _]
          tunnel: [w358 w376] -> w354
          tunnel: w353 -> [w357 w376]
          frame False {
            w372 = "Camera"
            w375 = FALSE ("Visible")
            n225 = local read "Camera Settings"() -> (w364:T2)
            n226 = Index Array(array=w365) -> (element=w368:cluster{string[]})  [unwired: 1 in]
            n227 = Unbundle(w364) -> ("Frame Rate"=w363:i32, "Compression"=w362:i32, "Size"=w366:u16)
            n228 = Unbundle(w368) -> (w367:string[])
            n229 = Index Array(array=w367, index=w366) -> (element=w361:string)
            n230 = call-poly <vilib>:"Write Key.vi"("section"=w372, "value"=w361, "key"="Size", "refnum"=w357) -> ("refnum out"=w374:T14)  [unwired: 2 in, 5 out]
            n231 = call-poly <vilib>:"Write Key.vi"("section"=w372, "value"=w363, "key"="FrameRate", "refnum"=w374) -> ("refnum out"=w373:T14)  [unwired: 1 in, 6 out]
            n232 = local write "DB Camera Config"(w375) -> ()
            n233 = property on="Camera Settings" class="Clust (strict)"("Visible"=w375) -> ()  [unwired: 2 in, 2 out]
            n234 = call-poly <vilib>:"Write Key.vi"("section"=w372, "value"=w362, "key"="Compression", "refnum"=w373) -> ("refnum out"=w359:T14)  [unwired: 1 in, 6 out]
            n235 = call <vilib>:"Close Config Data.vi"("refnum"=w359) -> ("file path"=w360:path)  [unwired: 2 in, 8 out]
            n236 = call <vilib>:"Open Config Data.vi"("configuration file path"=w360) -> ("refnum"=w358:T14)  [unwired: 8 in, 2 out]
          }
          frame True {
            n237 = property on="Camera Settings" class="Clust (strict)"("Visible"=TRUE) -> ()  [unwired: 2 in, 2 out]
          }
        }
      }
      event "Camera Settings": Value Change {
        n238 = event-data() -> ("NewVal"=w389:T2)  [unwired: 1 in]
        n239 = Index Array(array=w385) -> (element=w384:cluster{string[]})  [unwired: 1 in]
        n240 = Unbundle(w389) -> ("Frame Rate"=w380:i32, "Compression"=w379:i32, "Size"=w382:u16)
        n241 = Unbundle(w384) -> (w383:string[])
        n242 = Index Array(array=w383, index=w382) -> (element=w381:string)
        n243 = Format Into String(format string="%s   %dfps   %d%%", w381, w380, w379) -> (resulting string=w386:string)  [unwired: 2 in, 1 out]
        n244 = Build Array(w386) -> (w387:string[])
        n245 = property on="DB Camera Config" class="Bool (strict)"("Strings [4]"=w387) -> ()  [unwired: 2 in, 2 out]
      }
      event "Motor.Enable": Value Change {
        n246 = event-data() -> ("NewVal"=w395:bool)  [unwired: 1 in]
        n247 = Unbundle("Motor") -> ("Value"=w394:dbl)  [unwired: 1 out]
        n248 = Select(t=w394, s=w395, f=0.0) -> (s? t:f=w392:dbl)
        n249 = call <vilib>:"NT Write Number.vi"("Numeric"=w392, "Name"=w391) -> ()  [unwired: 9 in, 1 out]
      }
      event "Test Slider": Value Change {
        n250 = event-data() -> ("NewVal"=w398:dbl)  [unwired: 1 in]
        n251 = call <vilib>:"NT Write Number.vi"("Numeric"=w398, "Name"=w399) -> ()  [unwired: 9 in, 1 out]
      }
      event "On/Off": Value Change {
        n252 = event-data() -> ("NewVal"=w403:bool)  [unwired: 1 in]
        n253 = Boolean To (0,1)(Boolean=w403) -> (0, 1=w402:i16)
        n254 = call <vilib>:"NT Write Number.vi"("Numeric"=w402, "Name"=w401) -> ()  [unwired: 9 in, 1 out]
      }
      event "Rev/Fwd": Value Change {
        n255 = event-data() -> ("NewVal.Forward"=w411:bool, "NewVal.Reverse"=w410:bool)  [unwired: 1 in]
        n256 = Boolean To (0,1)(Boolean=w411) -> (0, 1=w407:i16)
        n257 = Boolean To (0,1)(Boolean=w410) -> (0, 1=w409:i16)
        n258 = Negate(x=w409) -> (-x=w408:i16)
        n259 = Add(x=w407, y=w408) -> (x+y=w406:i16)
        n260 = call <vilib>:"NT Write Number.vi"("Numeric"=w406, "Name"=w405) -> ()  [unwired: 9 in, 1 out]
      }
      event "Test Ring": Value Change {
        n261 = event-data() -> ("NewVal"=w415:u16)  [unwired: 1 in]
        n262 = property on="Test Ring" class="Ring (strict)"() -> ("Strings []"=w416:string[])  [unwired: 2 in, 2 out]
        n263 = Index Array(array=w416, index=w415) -> (element=w414:string)
        n264 = call <vilib>:"NT Write String.vi"("String"=w414, "Name"=w413) -> ()  [unwired: 9 in, 1 out]
      }
      event "Rec Mode": Value Change {
        # "Update globals for recording mode and path to read log from.\nClear when logging and let NetworkTables set path for vision to\nuse."
        n265 = event-data() -> ("NewVal"=w426:enum32{"Stop", "Record", "Playback"})  [unwired: 1 in]
        n266 = global write "WPI_DashboardLogging Global.vi" "Logging Filename"(path "") -> ()
        n267 = global write "WPI_DashboardLogging Global.vi" "Recording"(w426) -> ()
        n268 = case shown="\"Stop\", \"Record\"" w426 {
          tunnel: w425 -> [_ w428 w436]
          tunnel: [_ _ w435] -> w422
          tunnel: [_ _ w434] -> _
          tunnel: w420 -> [_ _ w432]
          tunnel: cluster{i32, i32} {-250, 170} -> [_ _ w431]
          tunnel: [_ _ T16 {"Image Size"=TRUE, "Image Type"=TRUE, "Pixel Value"=TRUE, "ROI Information"=TRUE, "Zoom Factor"=FALSE} ("Image Information Shown:All Elements")] -> w418
          tunnel: [_ _ TRUE ("Zoom Factor")] -> w417
          frame Default {
          }
          frame "Stop", "Record" {
            # "Place Window too"
            n269 = invoke class="VI" method="FP.Close"(reference=w428) -> (reference out=w427:refnum<vi>)  [unwired: 2 in, 2 out]
            n270 = invoke class="VI" method="Abort VI"(reference=w427) -> ()  [unwired: 2 in, 3 out]
          }
          frame "Playback" {
            n271 = call "Open Playback Panel.vi"("Offset"=w431, "DB VI Ref"=w432, "Playback in"=w436) -> ("Playback out"=w433:refnum<vi>)  [unwired: 8 in]
            n272 = register-events(w433) -> (reference out=w435:refnum<event-registration>, error out=w434:errorcluster)  [unwired: 2 in]
          }
        }
        n273 = property on="Camera Image" class="ImageControl"("Image Information Shown"=w418, "Image Information Visible"=w417) -> ()  [unwired: 2 in, 2 out]
        n274 = call <vilib>:"WPI_DashboardNT Log FieldName Cache.vi"("Operation"=enum16{"Lookup/Add", "Index", "Clear"}."Clear") -> ()  [unwired: 8 in, 3 out]
      }
      event Panel Close {
        w437 = enum32{"Stop", "Record", "Playback"}."Stop" ("Rec Mode")
        n275 = event-data() -> ()  [unwired: 1 in, 4 out]
        n276 = local write "Rec Mode"(w437) -> ()
        n277 = global write "WPI_DashboardLogging Global.vi" "Recording"(w437) -> ()
      }
      event Panel Close {
        # "Abort playback window and ourself"
        n278 = event-data() -> ()  [unwired: 1 in, 4 out]
        n279 = invoke class="VI" method="FP.Close"(reference=w442) -> (reference out=w441:refnum<vi>)  [unwired: 2 in, 2 out]
        n280 = invoke class="VI" method="Abort VI"(reference=w441) -> (error out=w440:errorcluster)  [unwired: 2 in, 2 out]
        n281 = invoke class="VI" method="Abort VI"(error in=w440) -> ()  [unwired: 2 in, 3 out]
      }
    }
  }
  n282 = property on="On/Off" class="Bool (strict)"("Visible"=w25) -> ()  [unwired: 2 in, 2 out]
  n283 = property on="Motor" class="Clust (strict)"("Visible"=w25) -> ()  [unwired: 2 in, 2 out]
  n284 = property on="Progress" class="Clust (strict)"("Visible"=w25) -> ()  [unwired: 2 in, 2 out]
  n285 = property on="Test Ring" class="Ring (strict)"("Visible"=w25) -> ()  [unwired: 2 in, 2 out]
  n286 = property on="Rev/Fwd" class="Clust (strict)"("Visible"=w25) -> ()  [unwired: 2 in, 2 out]
  n287 = local write "DB Camera Config"(w25) -> ()
  n288 = property on="Camera Settings" class="Clust (strict)"("Visible"=w25) -> ()  [unwired: 2 in, 2 out]
  n289 = global write "WPI_DashboardLogging Global.vi" "Recording"(w8) -> ()
  n290 = local write "Rec Mode"(w8) -> ()
